vi "Create Publish Topic Policy.vi"(8 "error in (no error)":errorcluster, 10 "Role Name":string, 11 "Topic in":refnum<class "Topic.lvclass">) -> (0 "error out":errorcluster, 3 "Topic out":refnum<class "Topic.lvclass">)   [LabVIEW 2015, in "NI_AWS_SNS.lvlib" / "Topic.lvclass"]
uses:
  Topic.lvclass
  Core/ARN/ARN.lvclass/ARN.ctl
  Core/HTTP Request/HTTP Request.lvclass/HTTP Request.ctl
  Core/ARN/Read ARN.vi
  Core/HTTP Request/Read Credentials.vi
  IAM/IAM Session/IAM Session.lvclass
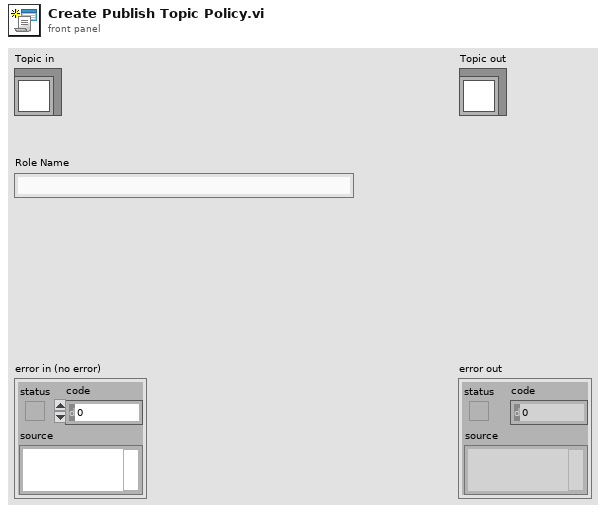
[diagram p1: front panel]
types:
  T1 = typedef "NI_AWS_Core.lvlib/HTTP Request.lvclass/AWS Credentials.ctl" = cluster{"Access Key":string, "Secret Key":string}
  T2 = typedef "NI_AWS_IAM.lvlib/Policy.ctl" = cluster{"Name":string, "Default Version ID":string, "ID":string, "Path":string, "ARN":string, "Attachment Count":i32, "Creation Date":string, "Last Updated Date":string}
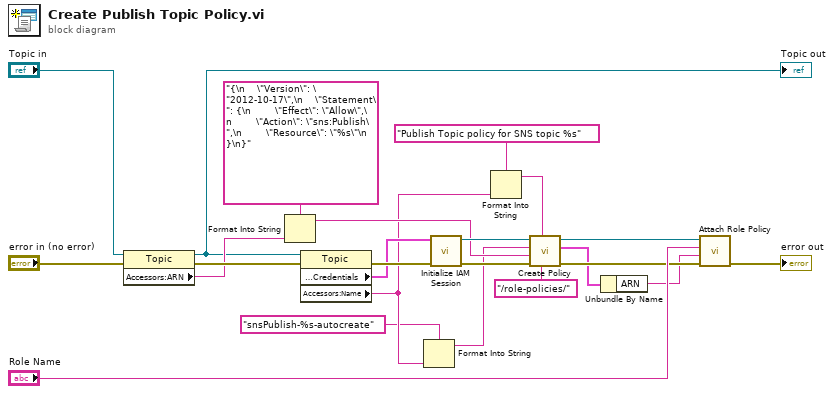
[diagram p0: block diagram]
diagram:
  n1 = property class="Topic"(reference="Topic in", error in="error in (no error)") -> (reference out=w1:refnum<class "Topic.lvclass">, error out=w19:errorcluster, "Accessors:ARN"=w2:string)
  "Topic out" <- w1
  n2 = Format Into String(format string="{\n    \"Version\": \"2012-10-17\",\n    \"Statement\": {\n        \"Effect\": \"Allow\",\n        \"Action\": \"sns:Publish\",\n        \"Resource\": \"%s\"\n    }\n}", w2) -> (resulting string=w6:string)  [unwired: 2 in, 1 out]
  n3 = property class="Topic"(reference=w1, error in=w19) -> (error out=w18:errorcluster, "Accessors:Credentials"=w17:T1, "Accessors:Name"=w5:string)  [unwired: 1 out]
  n4 = Format Into String(format string="snsPublish-%s-autocreate", w5) -> (resulting string=w3:string)  [unwired: 2 in, 1 out]
  n5 = call "Initialize IAM Session.vi"("error in (no error)"=w18, "AWS Credentials"=w17) -> ("error out"=w16:errorcluster, "IAM Session"=w15:refnum<class "IAM Session.lvclass">)  [unwired: 8 in]
  n6 = Format Into String(format string="Publish Topic policy for SNS topic %s", w5) -> (resulting string=w11:string)  [unwired: 2 in, 1 out]
  n7 = call "Create Policy.vi"("Path"="/role-policies/", "Description"=w11, "error in (no error)"=w16, "Document"=w6, "Name"=w3, "IAM Session in"=w15) -> ("error out"=w14:errorcluster, "Created Policy"=w9:T2, "IAM Session out"=w13:refnum<class "IAM Session.lvclass">)  [unwired: 3 in]
  n8 = Unbundle By Name(w9) -> ("ARN"=w8:string)
  n9 = call "Attach Role Policy.vi"("error in (no error)"=w14, "Policy ARN"=w8, "Role Name"="Role Name", "IAM Session in"=w13) -> ("error out"=→"error out":errorcluster)  [unwired: 6 in, 1 out]
